vi "Channel Mng Performance Test.vi"() -> ()   [LabVIEW 2021]
uses:
  CIFChannels/Typedef/Direction.ctl
  CIFTag/Double/CIFTagDouble.lvclass
  D:/dev/CIF-LVCore/src/Channels/CIFChannels/CIFChannels.lvclass
  <vilib>/Platform/TimedLoop/XDataNode/timing_clust.ctl
  <vilib>/Platform/TimedLoop/XDataNode/nitl_modes.ctl
  <vilib>/Platform/TimedLoop/XDataNode/wakeup.ctl
  CIFChannelMng.lvclass
  CIFChannels/CIFChannels.lvclass/CIFChannels.ctl
  CIFChannelMng.lvclass/CIFChannelMng.ctl
  7d13c5b7-0b44-4ab4-8a6c-0bcd63b70b59.vi
  c0ba1b46-a5a0-42bd-afb3-2f6832d2a88c.vi
  6a1b8880-d4c2-444f-a4b2-811244e6db06.vi
  10e1b524-69ef-478e-ae98-36060d5eb0d6.vi
  332321e3-b478-4438-b8ac-43cf378b23bb.vi
  <vilib>/CIFChannels/SubVIs/Add Error.vi
  7d13c5b7-0b44-4ab4-8a6c-0bcd63b70b59.vi/c28b0ead-42ad-4072-80a2-aca7f2bd7ce3.vi
  <vilib>/CIFChannels/SubVIs/CIFServices Fill In Error Info Ex.vi
  <vilib>/CIFChannels/SubVIs/Get dll Path.vi
  c0ba1b46-a5a0-42bd-afb3-2f6832d2a88c.vi/4bc1c15b-36ab-481f-b8dd-c64075ce723a.vi
  c0ba1b46-a5a0-42bd-afb3-2f6832d2a88c.vi/d83cb72b-7713-41fc-a3d1-682de79cf574.vi
  6a1b8880-d4c2-444f-a4b2-811244e6db06.vi/c28b0ead-42ad-4072-80a2-aca7f2bd7ce3.vi
  10e1b524-69ef-478e-ae98-36060d5eb0d6.vi/c28b0ead-42ad-4072-80a2-aca7f2bd7ce3.vi
  10e1b524-69ef-478e-ae98-36060d5eb0d6.vi/219d0231-d98b-4193-b5cc-84f90e3c9091.vi
  332321e3-b478-4438-b8ac-43cf378b23bb.vi/c28b0ead-42ad-4072-80a2-aca7f2bd7ce3.vi
  332321e3-b478-4438-b8ac-43cf378b23bb.vi/219d0231-d98b-4193-b5cc-84f90e3c9091.vi
  CIFCore/Common/Utilities/Add Error.vi
  CIFChannels/Accessors/Read Name.vi
  CIFChannels/Accessors/Read Custom Config Data.vi
  CIFChannels/Accessors/Read Type.vi
  CIFChannels/Accessors/Read Direction.vi
  Utilities/Get Channel Index by Name.vi
  CIFChannels/Accessors/Read Channel State.vi
  Utilities/Remove Channel by Index.vi
  <vilib>/CIFChannels/SubVIs/Append Error Location.vi
  CIFCore/Common/Utilities/Append Error Location.vi
  CIFChannels/Accessors/Write Channel State.vi
  <vilib>/Platform/TimedLoop/XDataNode/XDataNode.xnode
  CIFChannels/CIFChannels.lvclass
  <vilib>/Platform/TimedLoop/XDataNode/XDNodeRunTimeDep.lvlib
  <vilib>/CIFChannels/CIFChannelCore.lvlib
panel:
  out "avg dbl channel":dbl
  out "max dbl channel":dbl
  out "avg raw channel":dbl
  out "max raw channel":dbl
  out "pass":bool
  out "error out":errorcluster
  # "This test should be run on RT.  It stresses the communications by constantly creating resource contraints with the low priority sender and the high priority loop. On Windows the priority of the loops cannot be set."
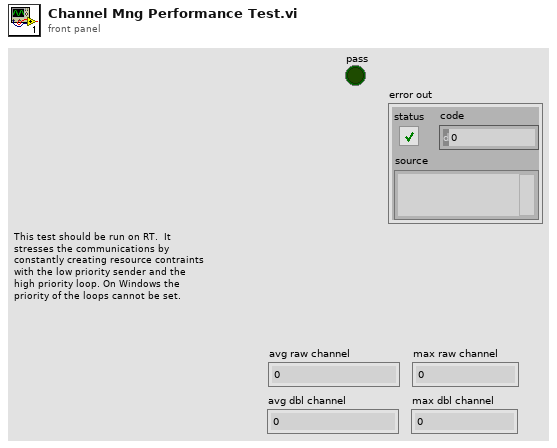
[diagram p1: front panel]
types:
  T1 = typedef "CIFChannels.lvclass/Direction.ctl" = enum16{"Publisher", "Subscriber"}
  T2 = typedef "XDNodeRunTimeDep.lvlib/timing_clust.ctl" = cluster{"Expected End [f-1]":u64, "Actual End [f-1]":u64, "Finished Late? [f-1]":bool, "Expected End [i-1]":u64, "Actual End [i-1]":u64, "Finished Late? [i-1]":bool, "Expected Start [i]":u64, "Actual Start [i]":u64, "Expected Start [f]":u64, "Actual Start [f]":u64, "Source Name":string, "Structure Name":string, "Period":i64, "Deadline":i64, "Offset":i64, "Start":i64, "Priority":i32, "Timeout":i32, "Mode":T3, "Wakeup Reason":T4, "Error":errorcluster, "Source Type":string, "Secondary Source Type":string, "Global End Time":u64, "Global Start Time":u64, "Frame Duration":u64, "Iteration Duration":u64, "Assigned CPU":i32, "I/O Scan Engine Mode":u32}
  T3 = typedef "XDNodeRunTimeDep.lvlib/nitl_modes.ctl" = enum32{"No Change", "Process missed periods, maintain original phase", "Discard missed periods, maintain original phase", "Process missed periods, ignore original phase", "Discard missed periods, ignore original phase"}
  T4 = typedef "XDNodeRunTimeDep.lvlib/wakeup.ctl" = enum32{"Normal", "Aborted", "Asynchronous wakeup", "Timing source error", "Timed loop error", "Timeout"}
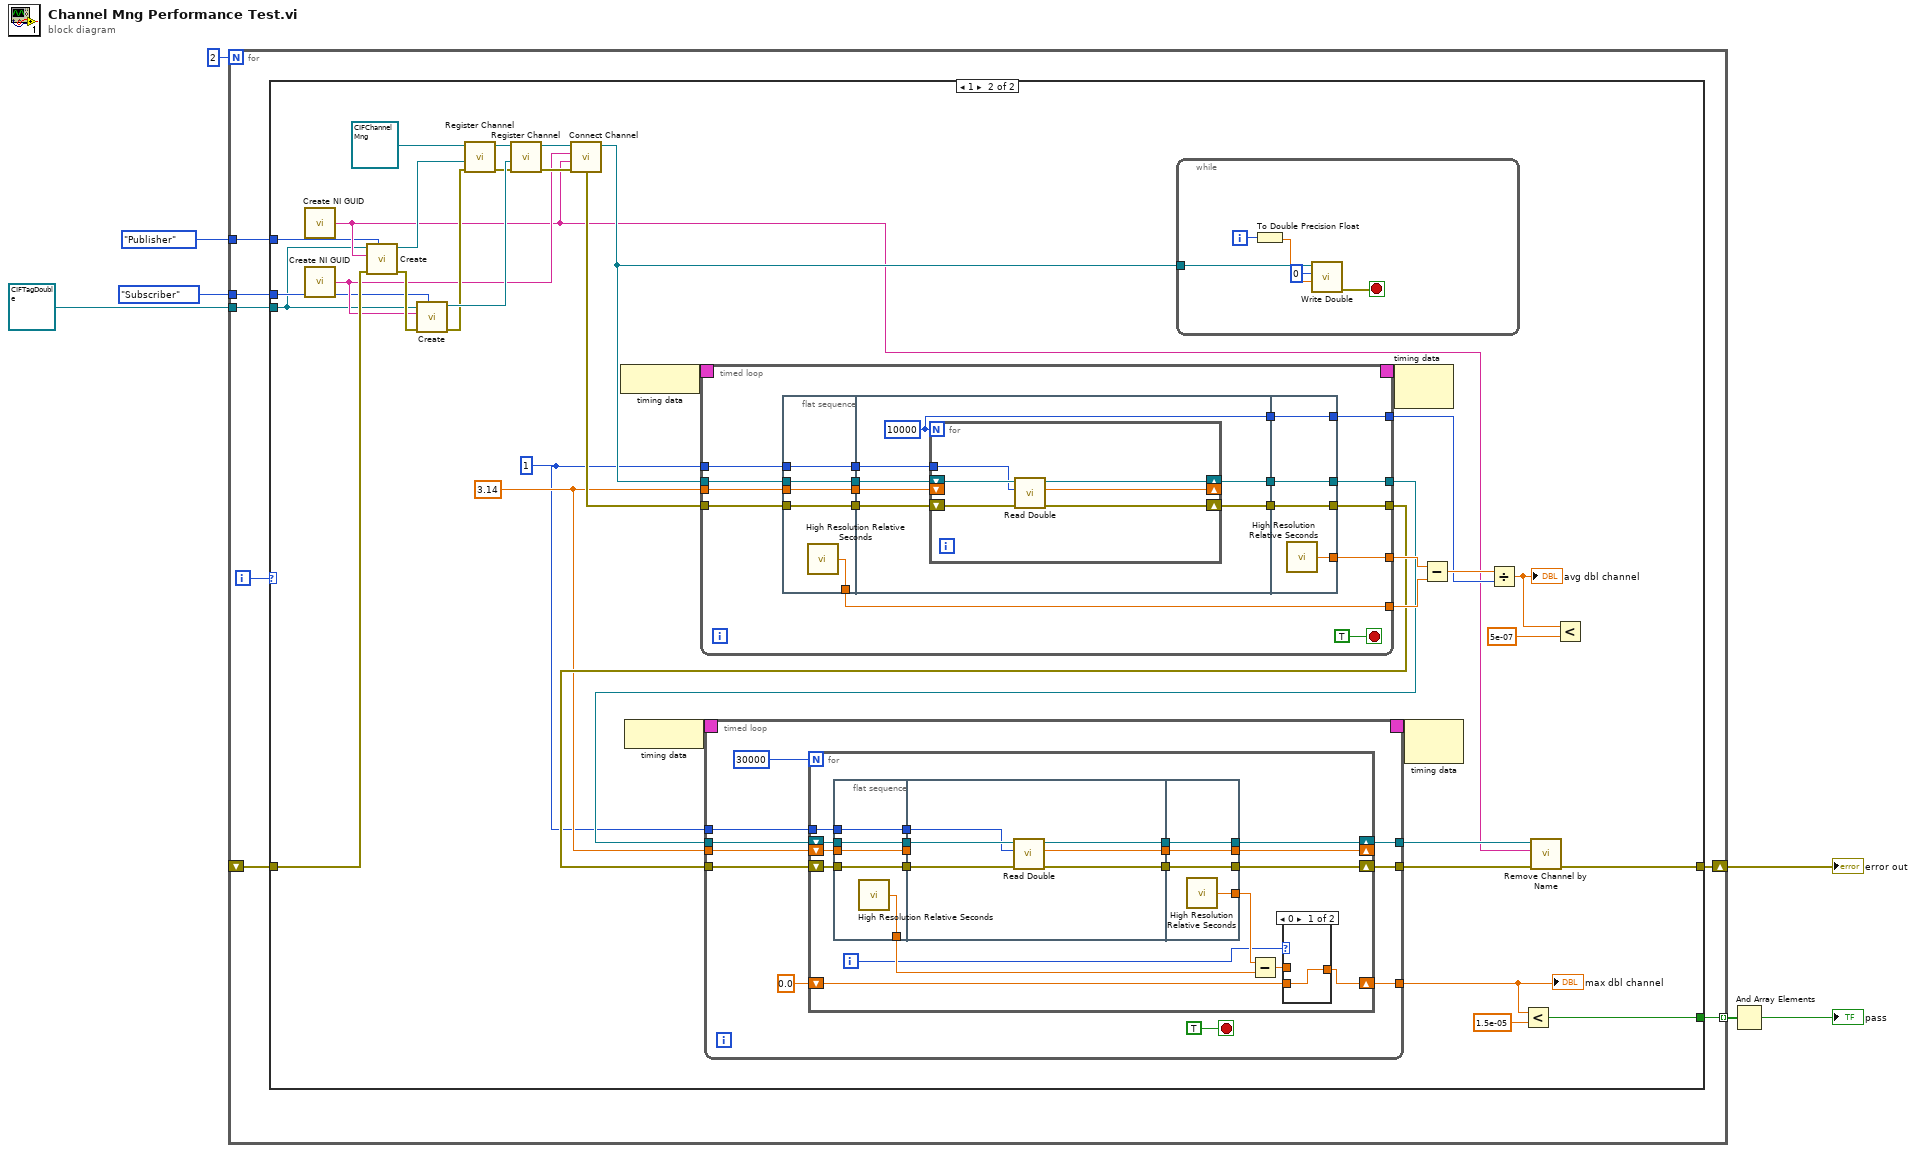
[diagram p0: block diagram]
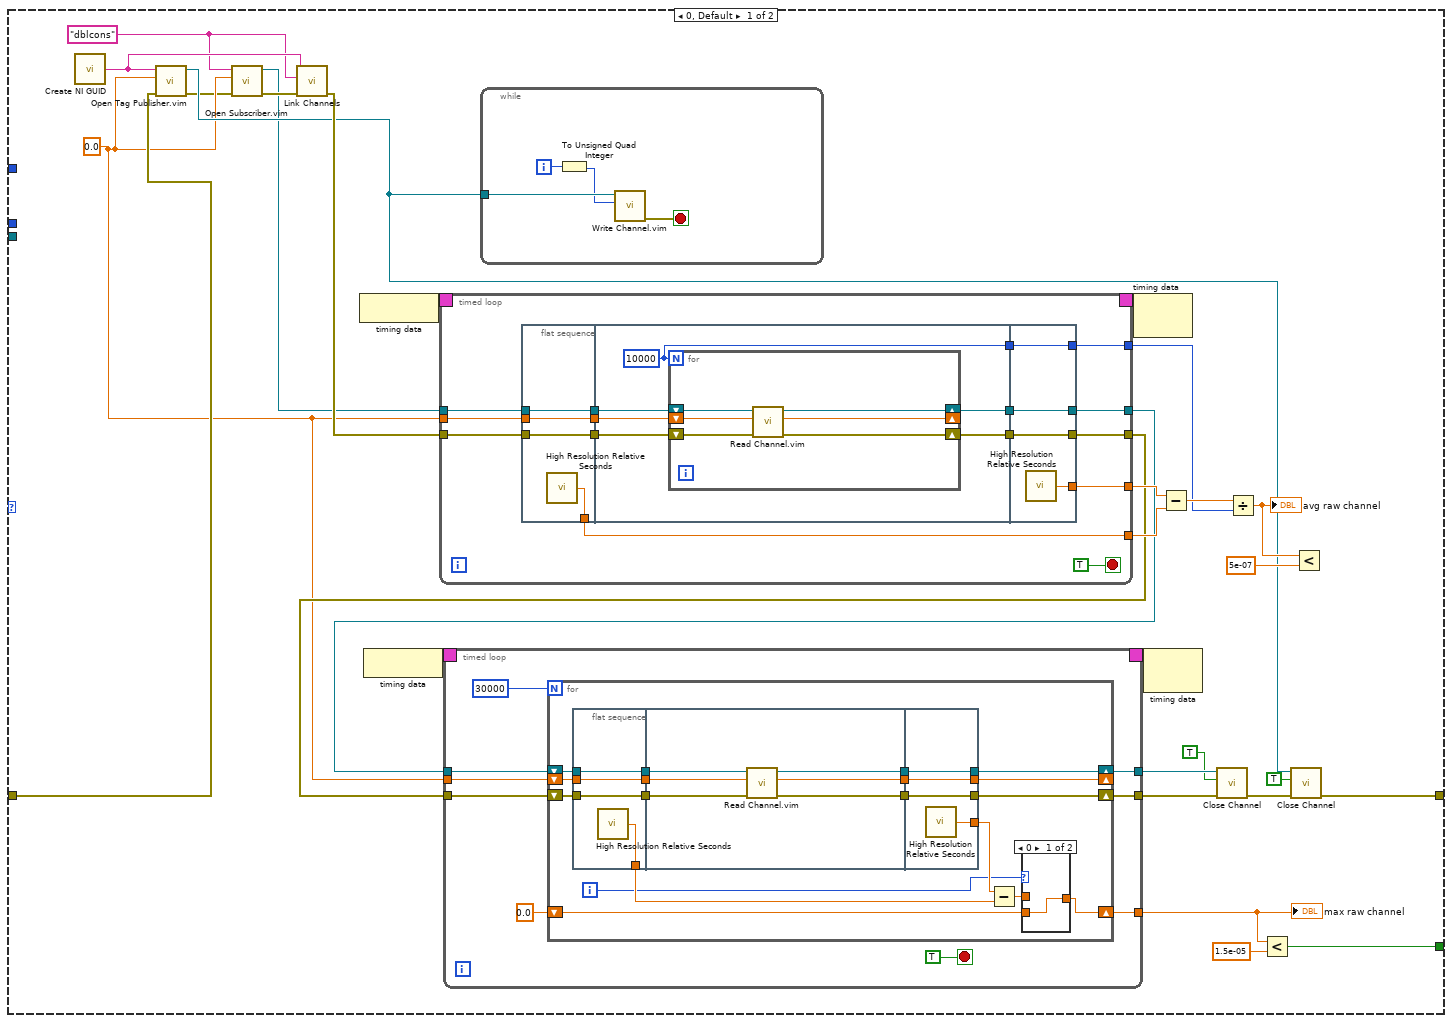
[diagram p2: hidden frame]
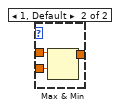
[diagram p3: hidden frame]
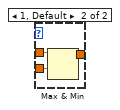
[diagram p4: hidden frame]
diagram:
  n1 = for {
    N: 2 -> [_]
    tunnel: [w14] -> w5 mode=indexing
    shift-right: [w13] -> w7
    shift-left: _ -> [w11]
    tunnel: Direction."Publisher" ("Direction") -> [w10]
    tunnel: Direction."Subscriber" ("Direction") -> [w9]
    tunnel: refnum<class "CIFTagDouble.lvclass"> refnum ("CIFTag in") -> [w8]
    i -> [w12]
    n2 = case shown="1" w12 {
      tunnel: [w30 w159] -> w14
      tunnel: [w23 w142] -> w13
      tunnel: w11 -> [w28 w149]
      tunnel: w10 -> [_ w140]
      tunnel: w9 -> [_ w139]
      tunnel: w8 -> [_ w138]
      frame 0, Default {
        w17 = "dblcons" ("Channel Name")
        w19 = 0.0
        n3 = call <vilib>:"Create NI GUID.vi"() -> ("NI GUID"=w21:string)
        n4 = call "Open Tag Publisher.vim"("error in"=w28, "Input Type"=w19, "Channel Name"=w21) -> ("error out"=w18:errorcluster, "CIF Channel"=w22:refnum<k21>)  [unwired: 7 in]
        n5 = call "Open Subscriber.vim"("error in"=w18, "Input Type"=w19, "Channel Name"=w17) -> ("error out"=w16:errorcluster, "CIF Channel"=w15:refnum<k21>)  [unwired: 7 in]
        n6 = call <vilib>:"Link Channels.vi"("error in"=w16, "Consumer Channel Name"=w17, "Producer Channel Name"=w21) -> ("error out"=w29:errorcluster)  [unwired: 8 in]
        n7 = node-c288() -> (w44:T2)
        n8 = node-c288() -> (w42:T2)
        n9 = timed-loop {
          timing: w44 -> [_]
          timing-out: [_] -> w43
          tunnel: w15 -> [w112]
          tunnel: w29 -> [w111]
          tunnel: [w107] -> w36
          tunnel: [w105] -> w35
          tunnel: [w103] -> w40
          tunnel: [w102] -> w39
          tunnel: [w101] -> w37
          tunnel: w19 -> [w99]
          stop <- TRUE stop-if-true
          n10 = flat-sequence {
            tunnel: w111 -> [w115]
            tunnel: w112 -> [w116]
            tunnel: [w116] -> w109
            tunnel: [w115] -> w108
            tunnel: [w114] -> w102
            tunnel: w99 -> [w113]
            tunnel: [w113] -> w98
            tunnel: w109 -> [w122]
            tunnel: w108 -> [w121]
            tunnel: [w120] -> w106
            tunnel: [w119] -> w104
            tunnel: [w118] -> w100
            tunnel: w98 -> [w117]
            tunnel: [w132] -> w107
            tunnel: w106 -> [w132]
            tunnel: [w131] -> w105
            tunnel: w104 -> [w131]
            tunnel: [w130] -> w103
            tunnel: [w129] -> w101
            tunnel: w100 -> [w129]
            frame #0 {
              n11 = call <vilib>:"High Resolution Relative Seconds.vi"() -> ("relative seconds"=w114:dbl)
            }
            frame #1 {
              w118 = 10000
              n12 = for {
                N: w118 -> [_]
                shift-right: [w125] -> w120
                shift-left: w122 -> [w128]
                shift-right: [w124] -> w119
                shift-left: w121 -> [w123]
                shift-right: [w126] -> _
                shift-left: w117 -> [w127]
                n13 = call "Read Channel.vim"("error in"=w123, "Data in"=w127, "CIF Channel in"=w128) -> ("error out"=w124:errorcluster, "Data out"=w126:dbl, "CIF Channel out"=w125:refnum<k21>)  [unwired: 5 in, 1 out]
              }
            }
            frame #2 {
              n14 = call <vilib>:"High Resolution Relative Seconds.vi"() -> ("relative seconds"=w130:dbl)
            }
          }
        }
        n15 = timed-loop {
          timing: w42 -> [_]
          timing-out: [_] -> w41
          tunnel: w36 -> [w57]
          tunnel: w35 -> [w56]
          tunnel: [w54] -> w26
          tunnel: [w53] -> w27
          tunnel: w19 -> [w52]
          tunnel: [w49] -> w32
          stop <- TRUE stop-if-true
          n16 = for {
            N: 30000 -> [_]
            shift-right: [w69] -> w54
            shift-left: w57 -> [w71]
            shift-right: [w68] -> w53
            shift-left: w56 -> [w70]
            shift-right: [w62] -> w49
            shift-left: 0.0 -> [w63]
            shift-right: [w61] -> _
            shift-left: w52 -> [w67]
            i -> [w59]
            n17 = flat-sequence {
              tunnel: w70 -> [w82]
              tunnel: w71 -> [w83]
              tunnel: [w83] -> w75
              tunnel: [w82] -> w74
              tunnel: [w81] -> w65
              tunnel: w67 -> [w80]
              tunnel: [w80] -> w73
              tunnel: w75 -> [w89]
              tunnel: w74 -> [w85]
              tunnel: [w88] -> w72
              tunnel: w73 -> [w87]
              tunnel: [w86] -> w60
              tunnel: [w84] -> w58
              tunnel: [w93] -> w69
              tunnel: w72 -> [w93]
              tunnel: [w92] -> w68
              tunnel: [w91] -> w66
              tunnel: [w90] -> w61
              tunnel: w60 -> [w90]
              tunnel: w58 -> [w92]
              frame #0 {
                n18 = call <vilib>:"High Resolution Relative Seconds.vi"() -> ("relative seconds"=w81:dbl)
              }
              frame #1 {
                n19 = call "Read Channel.vim"("error in"=w85, "Data in"=w87, "CIF Channel in"=w89) -> ("error out"=w84:errorcluster, "Data out"=w86:dbl, "CIF Channel out"=w88:refnum<k21>)  [unwired: 5 in, 1 out]
              }
              frame #2 {
                n20 = call <vilib>:"High Resolution Relative Seconds.vi"() -> ("relative seconds"=w91:dbl)
              }
            }
            n21 = Subtract(x=w66, y=w65) -> (x-y=w64:dbl)
            n22 = case shown="0" w59 {
              tunnel: w64 -> [_ w79]
              tunnel: w63 -> [w76 w78]
              tunnel: [w76 w77] -> w62
              frame 0 {
              }
              frame 1, Default {
                n23 = Max & Min(x=w79, y=w78) -> (max(x,y)=w77:dbl)  [unwired: 1 out]
              }
            }
          }
        }
        "max raw channel" <- w32
        n24 = while {
          tunnel: w22 -> [w47]
          i -> [w48]
          stop <- w45 stop-if-true
          n25 = To Unsigned Quad Integer(1:w48) -> (0:w46:u64)
          n26 = call "Write Channel.vim"("Data in"=w46, "CIF Channel in"=w47) -> ("error out"=w45:errorcluster)  [unwired: 6 in, 3 out]
        }
        n27 = node-c288(w43) -> ()  [unwired: 1 out]
        n28 = node-c288(w41) -> ()  [unwired: 1 out]
        n29 = Subtract(x=w40, y=w39) -> (x-y=w38:dbl)
        n30 = call <vilib>:"Close Channel.vi"("error in"=w27, "Force Destroy? (F)"=TRUE, "CIF Channel"=w26) -> ("error out"=w25:errorcluster)  [unwired: 8 in]
        n31 = Divide(x=w38, y=w37) -> (x/y=w34:dbl)
        "avg raw channel" <- w34
        n32 = Less?(x=w32, y=1.5e-05) -> (x < y?=w30:bool)
        n33 = call <vilib>:"Close Channel.vi"("error in"=w25, "Force Destroy? (F)"=TRUE, "CIF Channel"=w22) -> ("error out"=w23:errorcluster)  [unwired: 8 in]
        n34 = Less?(x=w34, y=5e-07) -> ()  [unwired: 1 out]
      }
      frame 1 {
        w137 = 1 ("Channel Index")
        w146 = 3.14 ("Default Value")
        n35 = call <vilib>:"Create NI GUID.vi"() -> ("NI GUID"=w141:string)
        n36 = call <vilib>:"Create NI GUID.vi"() -> ("NI GUID"=w145:string)
        n37 = call-dynamic "Create.vi"("Direction"=w140, "error in (no error)"=w149, "Name"=w141, "CIFTag in"=w138) -> ("error out"=w154:errorcluster, "CIFTag out"=w153:refnum<class "CIFTagDouble.lvclass">)  [unwired: 6 in]
        n38 = call-dynamic "Create.vi"("Direction"=w139, "error in (no error)"=w154, "Name"=w145, "CIFTag in"=w138) -> ("error out"=w155:errorcluster, "CIFTag out"=w158:refnum<class "CIFTagDouble.lvclass">)  [unwired: 6 in]
        n39 = call "Register Channel.vi"("error in (no error)"=w155, "Channel"=w153, "CIFChannelMng in"=refnum<class "CIFChannelMng.lvclass"> refnum) -> ("error out"=w152:errorcluster, "CIFChannelMng out"=w151:refnum<class "CIFChannelMng.lvclass">)  [unwired: 7 in]
        n40 = call "Register Channel.vi"("error in (no error)"=w152, "Channel"=w158, "CIFChannelMng in"=w151) -> ("error out"=w157:errorcluster, "CIFChannelMng out"=w156:refnum<class "CIFChannelMng.lvclass">)  [unwired: 7 in]
        n41 = call "Connect Channel.vi"("error in (no error)"=w157, "Publisher Name"=w141, "Subscriber Name"=w145, "CIFChannelMng in"=w156) -> ("error out"=w148:errorcluster, "CIFChannelMng out"=w147:refnum<class "CIFChannelMng.lvclass">)  [unwired: 6 in]
        n42 = node-c288() -> (w173:T2)
        n43 = node-c288() -> (w171:T2)
        n44 = timed-loop {
          timing: w173 -> [_]
          timing-out: [_] -> w172
          tunnel: w147 -> [w248]
          tunnel: w148 -> [w247]
          tunnel: [w243] -> w165
          tunnel: [w241] -> w164
          tunnel: [w239] -> w169
          tunnel: [w238] -> w168
          tunnel: [w237] -> w166
          tunnel: w146 -> [w235]
          tunnel: w137 -> [w233]
          stop <- TRUE stop-if-true
          n45 = flat-sequence {
            tunnel: w247 -> [w252]
            tunnel: w248 -> [w253]
            tunnel: [w253] -> w245
            tunnel: [w252] -> w244
            tunnel: [w251] -> w238
            tunnel: w235 -> [w250]
            tunnel: [w250] -> w234
            tunnel: w233 -> [w249]
            tunnel: [w249] -> w232
            tunnel: w245 -> [w260]
            tunnel: w244 -> [w259]
            tunnel: [w258] -> w242
            tunnel: [w257] -> w240
            tunnel: [w256] -> w236
            tunnel: w234 -> [w255]
            tunnel: w232 -> [w254]
            tunnel: [w270] -> w243
            tunnel: w242 -> [w270]
            tunnel: [w269] -> w241
            tunnel: w240 -> [w269]
            tunnel: [w268] -> w239
            tunnel: [w267] -> w237
            tunnel: w236 -> [w267]
            frame #0 {
              n46 = call <vilib>:"High Resolution Relative Seconds.vi"() -> ("relative seconds"=w251:dbl)
            }
            frame #1 {
              w256 = 10000
              n47 = for {
                N: w256 -> [_]
                shift-right: [w265] -> w258
                shift-left: w260 -> [w266]
                shift-right: [w264] -> w257
                shift-left: w259 -> [w263]
                shift-right: [w262] -> _
                shift-left: w255 -> [_]
                tunnel: w254 -> [w261]
                n48 = call "Read Double.vi"("error in (no error)"=w263, "Channel Index"=w261, "CIFChannelMng in"=w266) -> ("error out"=w264:errorcluster, "Data"=w262:dbl, "CIFChannelMng out"=w265:refnum<class "CIFChannelMng.lvclass">)  [unwired: 5 in, 1 out]
              }
            }
            frame #2 {
              n49 = call <vilib>:"High Resolution Relative Seconds.vi"() -> ("relative seconds"=w268:dbl)
            }
          }
        }
        n50 = timed-loop {
          timing: w171 -> [_]
          timing-out: [_] -> w170
          tunnel: w165 -> [w188]
          tunnel: w164 -> [w187]
          tunnel: [w185] -> w144
          tunnel: [w184] -> w143
          tunnel: w146 -> [w183]
          tunnel: [w180] -> w161
          tunnel: w137 -> [w179]
          stop <- TRUE stop-if-true
          n51 = for {
            N: 30000 -> [_]
            shift-right: [w202] -> w185
            shift-left: w188 -> [w204]
            shift-right: [w201] -> w184
            shift-left: w187 -> [w203]
            shift-right: [w195] -> w180
            shift-left: 0.0 -> [w196]
            shift-right: [w194] -> _
            shift-left: w183 -> [w200]
            tunnel: w179 -> [w190]
            i -> [w192]
            n52 = flat-sequence {
              tunnel: w203 -> [w216]
              tunnel: w204 -> [w217]
              tunnel: [w217] -> w208
              tunnel: [w216] -> w207
              tunnel: [w215] -> w198
              tunnel: w200 -> [w214]
              tunnel: [w214] -> w206
              tunnel: w190 -> [w213]
              tunnel: [w213] -> w189
              tunnel: w208 -> [w222]
              tunnel: w207 -> [w223]
              tunnel: [w221] -> w205
              tunnel: w206 -> [_]
              tunnel: [w219] -> w193
              tunnel: [w220] -> w191
              tunnel: w189 -> [w218]
              tunnel: [w227] -> w202
              tunnel: w205 -> [w227]
              tunnel: [w226] -> w201
              tunnel: [w225] -> w199
              tunnel: [w224] -> w194
              tunnel: w193 -> [w224]
              tunnel: w191 -> [w226]
              frame #0 {
                n53 = call <vilib>:"High Resolution Relative Seconds.vi"() -> ("relative seconds"=w215:dbl)
              }
              frame #1 {
                n54 = call "Read Double.vi"("error in (no error)"=w223, "Channel Index"=w218, "CIFChannelMng in"=w222) -> ("error out"=w220:errorcluster, "Data"=w219:dbl, "CIFChannelMng out"=w221:refnum<class "CIFChannelMng.lvclass">)  [unwired: 5 in, 1 out]
              }
              frame #2 {
                n55 = call <vilib>:"High Resolution Relative Seconds.vi"() -> ("relative seconds"=w225:dbl)
              }
            }
            n56 = Subtract(x=w199, y=w198) -> (x-y=w197:dbl)
            n57 = case shown="0" w192 {
              tunnel: w197 -> [_ w212]
              tunnel: w196 -> [w209 w211]
              tunnel: [w209 w210] -> w195
              frame 0 {
              }
              frame 1, Default {
                n58 = Max & Min(x=w212, y=w211) -> (max(x,y)=w210:dbl)  [unwired: 1 out]
              }
            }
          }
        }
        "max dbl channel" <- w161
        n59 = while {
          tunnel: w147 -> [w177]
          i -> [w178]
          stop <- w175 stop-if-true
          n60 = To Double Precision Float(number=w178) -> (double precision float=w176:dbl)
          n61 = call "Write Double.vi"("Data"=w176, "Channel Index"=0, "CIFChannelMng in"=w177) -> ("error out"=w175:errorcluster)  [unwired: 6 in, 2 out]
        }
        n62 = node-c288(w172) -> ()  [unwired: 1 out]
        n63 = node-c288(w170) -> ()  [unwired: 1 out]
        n64 = Subtract(x=w169, y=w168) -> (x-y=w167:dbl)
        n65 = Divide(x=w167, y=w166) -> (x/y=w163:dbl)
        "avg dbl channel" <- w163
        n66 = Less?(x=w161, y=1.5e-05) -> (x < y?=w159:bool)
        n67 = call "Remove Channel by Name.vi"("error in (no error)"=w143, "Channel Name"=w141, "CIFChannelMng in"=w144) -> ("error out"=w142:errorcluster)  [unwired: 7 in, 1 out]
        n68 = Less?(x=w163, y=5e-07) -> ()  [unwired: 1 out]
      }
    }
  }
  "error out" <- w7
  n69 = And Array Elements(Boolean array=w5) -> (logical AND=→"pass":bool)
